vi "Application Stop.vi"(7 "Command":enum16{"Read ", "Write "}(ring), 8 "error in (no error)":errorcluster, 11 "STOP":bool=TRUE) -> (0 "error out":errorcluster, 3 "STOP":bool=TRUE)   [LabVIEW 2018]
doc: "This Subvi usde for CSV Initialize ,Read, Write and close.\nIntilise case; we check File avaliblity in not found create csv file\nRead Case ; Read data from csv file"
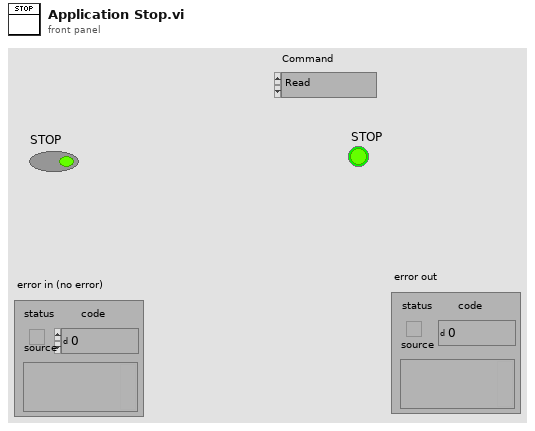
[diagram p1: front panel]
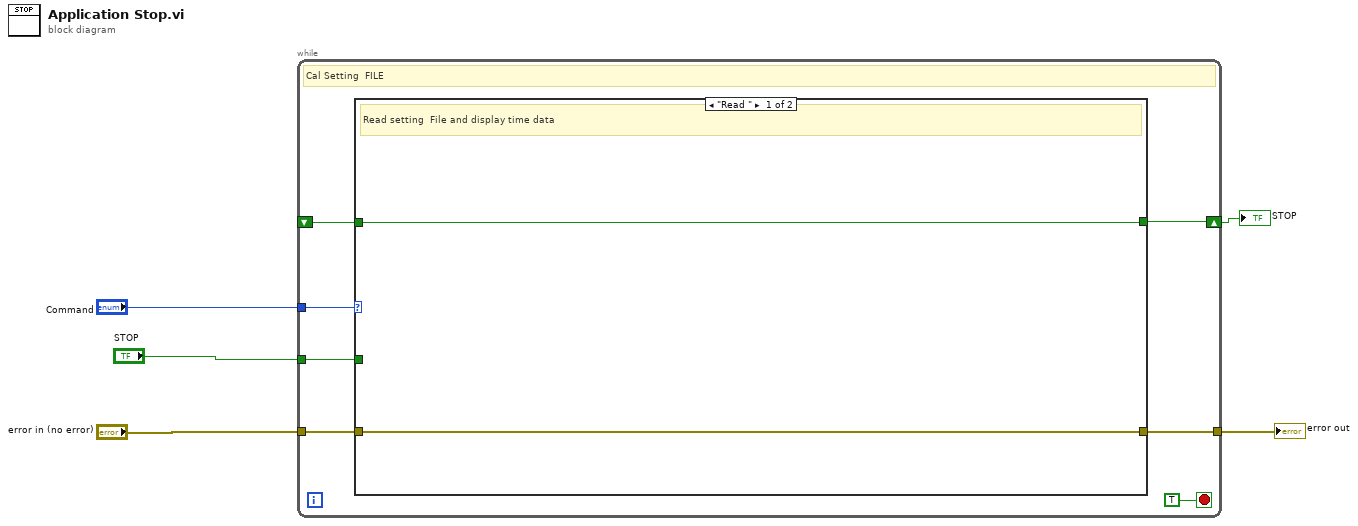
[diagram p0: block diagram]
diagram:
  n1 = while {
    shift-right: [w6] -> w1
    shift-left: _ -> [w8]
    tunnel: "Command" -> [w11]
    tunnel: "error in (no error)" -> [w10]
    tunnel: [w9] -> w5
    tunnel: "STOP" -> [w7]
    stop <- TRUE stop-if-true
    # "Cal Setting  FILE"
    n2 = case shown="\"Read \"" w11 {
      tunnel: w10 -> [w14 w16]
      tunnel: [w14 w16] -> w9
      tunnel: [w13 w15] -> w6
      tunnel: w8 -> [w13 _]
      tunnel: w7 -> [_ w15]
      frame "Read " {
        # "Read setting  File and display time data"
      }
      frame "Write " {
        # "Write Data in CSV file"
      }
    }
  }
  "error out" <- w5
  "STOP" <- w1
